vi "Get Columns.vi"(8 "error in (no error)":errorcluster, 10 "selected table path":string, 11 "Data.PG in":refnum<class "Data.PGSQL.lvclass">) -> (0 "error out":errorcluster, 1 "Column Paths":string[](array[string]), 2 "Column Names":string[](array[string]), 3 "Data.PG out":refnum<class "Data.PGSQL.lvclass">, 4 "Column Units":string[](array[string]))   [LabVIEW 2013, in "Data.PGSQL.lvclass"]
uses:
  Data.PGSQL.lvclass
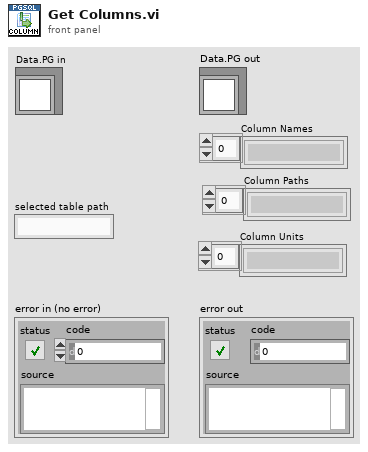
[diagram p1: front panel]
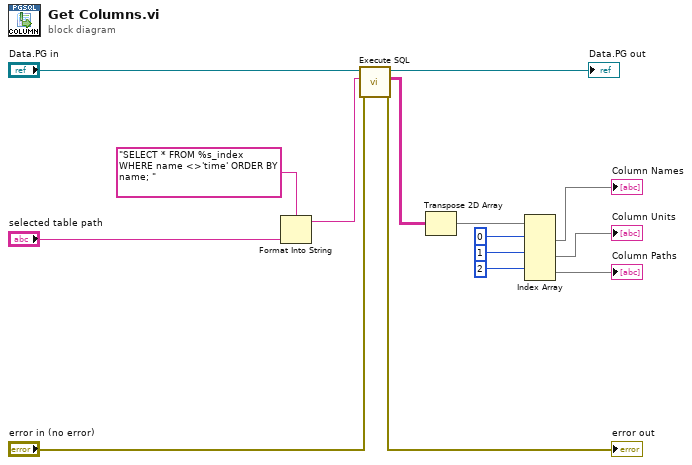
[diagram p0: block diagram]
diagram:
  n1 = Format Into String(format string="SELECT * FROM %s_index WHERE name <>'time' ORDER BY name; ", "selected table path") -> (resulting string=w8:string)  [unwired: 2 in, 1 out]
  n2 = call "Execute SQL.vi"("error in"="error in (no error)", "SQL"=w8, "Data.PG"="Data.PG in") -> ("error out"=→"error out":errorcluster, "Result"=w2:string[][], "Data.PG out"=→"Data.PG out":refnum<class "Data.PGSQL.lvclass">)  [unwired: 6 in]
  n3 = Transpose 2D Array(2D array=w2) -> (transposed array=w9:string[][])
  n4 = Index Array(array=w9, index (row) #1=0 ("index (row)"), index (row) #2=1 ("index (row)"), index (row) #3=2 ("index (row)")) -> (element #1=→"Column Names":string[], element #2=→"Column Units":string[], element #3=→"Column Paths":string[])  [unwired: 3 in]
